vi "subVI QCam Change Trigger Mode.vi"(3 "error in":errorcluster, 4 "trigger mode":T1(ring), 5 "cameraId In":u32) -> (0 "error out":errorcluster, 1 "trigger mode fbk":T1(ring), 2 "cameraId out":u32)   [LabVIEW 2012]
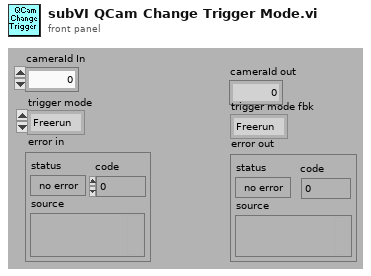
[diagram p1: front panel]
types:
  T1 = enum32{"Freerun", "Edge hi", "Edge low", "Pulse hi", "Pulse low", "Software"}
  T2 = enum32{"gain", "offset", "exposure", "binning", "horizontal binning", "vertical binning", "readout speed", "trigger type", "lcd filter", "cooler", "exposure red", "exposure blue", "image format", "roi x", "roi y", "roi width", "roi height", "reserved1", "shutter state", "reserved2", "sync-b out", "reserved3", "intensifier gain", "trigger delay", "camera mode", "normalized gain", "normalized intenifier gain DB", "doPostProcessing", "postProcessGainRed", "postProcessGainGreen", "postProcessGainBlue", "postProcessBayerAlgorithm", "postProcessImageFormat", "fan", "blackout mode", "high sensitivity", "Readout Port", "EM Gain", "open delay", "close delay", "clearing mode"}
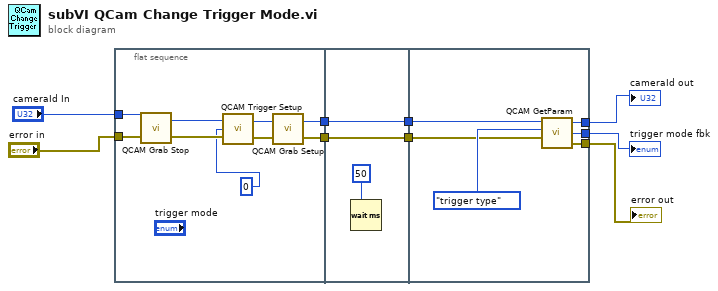
[diagram p0: block diagram]
diagram:
  n1 = flat-sequence {
    tunnel: [w14] -> w8
    tunnel: [w13] -> w6
    tunnel: "cameraId In" -> [w12]
    tunnel: "error in" -> [w11]
    tunnel: [w20] -> w9
    tunnel: w8 -> [w20]
    tunnel: [w19] -> w7
    tunnel: w6 -> [w19]
    tunnel: w9 -> [w27]
    tunnel: w7 -> [w25]
    tunnel: [w24] -> w3
    tunnel: [w23] -> w2
    tunnel: [w22] -> w1
    frame #0 {
      n2 = call "QCAM Grab Stop.vi"("error in (no error)"=w11, "cameraId"=w12) -> ("error out"=w17:errorcluster, "cameraId Out"=w18:u32)
      n3 = call "QCAM Trigger Setup.vi"("error in (no error)"=w17, "trigger mode"=0, "camera Id"=w18) -> ("error out"=w15:errorcluster, "camera Id out"=w16:u32)
      n4 = call <userlib>:"QCAM Grab Setup.vi"("error in (no error)"=w15, "cameraId"=w16) -> ("error out"=w13:errorcluster, "cameraId out"=w14:u32)
    }
    frame #1 {
      n5 = Wait (ms)(milliseconds to wait=50) -> ()  [unwired: 1 out]
    }
    frame #2 {
      n6 = call "QCAM GetParam.vi"("cameraId in"=w27, "parameter key"=T2."trigger type", "error in (no error)"=w25) -> ("cameraId out"=w24:u32, "value out"=w23:u32, "error out"=w22:errorcluster)  [unwired: 2 out]
    }
  }
  "trigger mode fbk" <- w2
  "cameraId out" <- w3
  "error out" <- w1
